vi "Joystick Sensitivity.vi"(9 "B":dbl, 10 "A":dbl, 11 "X":dbl) -> (3 "Y":dbl)   [LabVIEW 2015]
panel:
  out "Range":bool
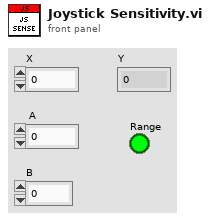
[diagram p1: front panel]
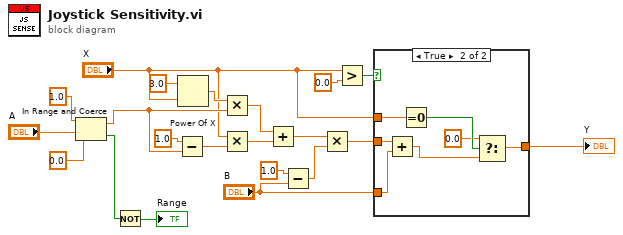
[diagram p0: block diagram]
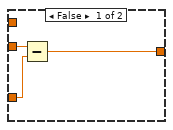
[diagram p2: hidden frame]
diagram:
  n1 = In Range and Coerce(upper limit=1.0, x="A", lower limit=0.0) -> (coerced(x)=w4:dbl, In Range?=w3:bool)
  n2 = Not(x=w3) -> (.not. x?=→"Range":bool)
  n3 = Subtract(x=1.0 ("y"), y=w4) -> (x-y=w10:dbl)
  n4 = Power Of X(1:"X", 2:3.0 ("y")) -> (0:w11:dbl)
  n5 = Multiply(x=w11, y=w4) -> (x*y=w13:dbl)
  n6 = Multiply(x="X", y=w10) -> (x*y=w12:dbl)
  n7 = Add(x=w13, y=w12) -> (x+y=w16:dbl)
  n8 = Subtract(x=1.0, y="B") -> (x-y=w15:dbl)
  n9 = Multiply(x=w16, y=w15) -> (x*y=w19:dbl)
  n10 = Greater?(x="X", y=0.0) -> (0:w18:bool)
  n11 = case shown="True" w18 {
    tunnel: w19 -> [w24 w31]
    tunnel: "B" -> [w23 w30]
    tunnel: [w22 w27] -> w21
    tunnel: "X" -> [_ w29]
    frame False {
      n12 = Subtract(x=w24, y=w23) -> (x-y=w22:dbl)
    }
    frame True {
      n13 = Add(x=w31, y=w30) -> (x+y=w26:dbl)
      n14 = Equal To 0?(x=w29) -> (x = 0?=w28:bool)
      n15 = Select(t=0.0, s=w28, f=w26) -> (s? t:f=w27:dbl)
    }
  }
  "Y" <- w21
